vi "waveSawtooth.vi"(3 "smoothing param":dbl, 4 "w":dbl, 5 "t":dbl) -> (0 "__square(x/2)":dbl, 1 "__triangle((2x-1)/4":dbl, 2 "sawtooth":dbl)   [LabVIEW 2017]
panel:
  # "https://mathematica.stackexchange.com/questions/38293/make-a-differentiable-smooth-sawtooth-waveform"
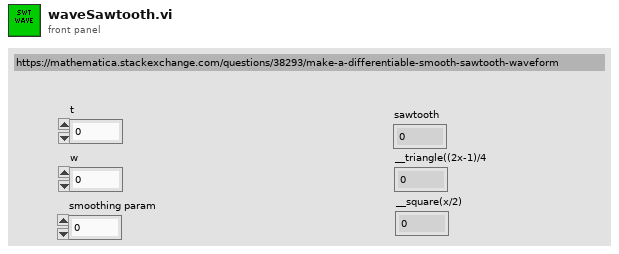
[diagram p1: front panel]
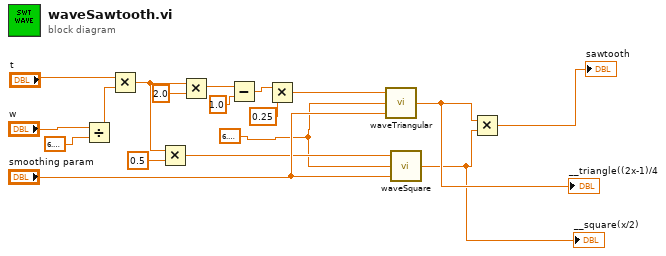
[diagram p0: block diagram]
diagram:
  w2 = 6.283185307179586
  n1 = Divide(x="w", y=6.283185307179586) -> (x/y=w3:dbl)
  n2 = Multiply(x="t", y=w3) -> (x*y=w7:dbl)
  n3 = Multiply(x=w7, y=0.5) -> (x*y=w15:dbl)
  n4 = Multiply(x=w7, y=2.0) -> (x*y=w9:dbl)
  n5 = Subtract(x=w9, y=1.0) -> (x-y=w8:dbl)
  n6 = Multiply(x=w8, y=0.25) -> (x*y=w13:dbl)
  n7 = call "waveTriangular.vi"("smoothing param"="smoothing param", "w"=w2, "t"=w13) -> ("y"=w12:dbl)
  "__triangle((2x-1)/4" <- w12
  n8 = call "waveSquare.vi"("smoothing param"="smoothing param", "w"=w2, "t"=w15) -> ("y"=w11:dbl)
  "__square(x/2)" <- w11
  n9 = Multiply(x=w12, y=w11) -> (x*y=→"sawtooth":dbl)
